vi "sub_log_fine-name.vi"() -> (3 "log path":string)   [LabVIEW 2019]
uses:
  logfile-name.vi
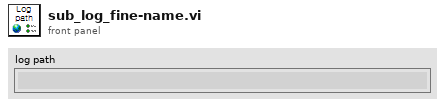
[diagram p1: front panel]
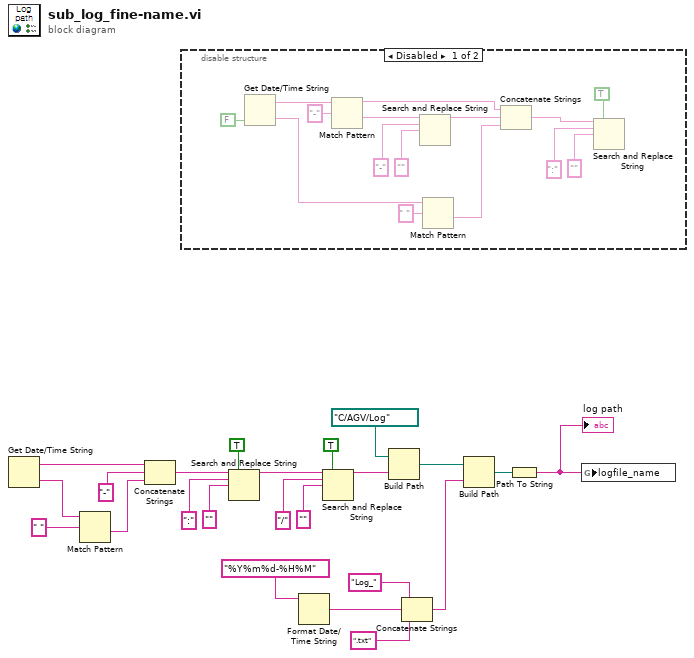
[diagram p0: block diagram]
diagram:
  n1 = Get Date/Time String() -> (date string=w11:string, time string=w17:string)  [unwired: 3 in]
  n2 = Match Pattern(string=w17, regular expression=" " ("정규식")) -> (after substring=w16:string)  [unwired: 1 in, 3 out]
  n3 = Concatenate Strings(w11, "-" ("정규식"), w16) -> (w12:string)
  n4 = disable-structure shown="Disabled" {
    frame Disabled {
      n5 = Get Date/Time String(want seconds? (F)=FALSE ("초 보이기? (거짓)")) -> (date string=w33:string, time string=w30:string)  [unwired: 2 in]
      n6 = Match Pattern(string=w33, regular expression="-" ("정규식")) -> (before substring=w24:string, after substring=w28:string)  [unwired: 1 in, 2 out]
      n7 = Search and Replace String(input string=w28, search string="-" ("검색 문자열"), replace string="" ("대체 문자열(\"\")")) -> (result string=w25:string)  [unwired: 5 in, 3 out]
      n8 = Match Pattern(string=w30, regular expression=" " ("정규식")) -> (after substring=w29:string)  [unwired: 1 in, 3 out]
      n9 = Concatenate Strings(w24, w25, w29) -> (w38:string)
      n10 = Search and Replace String(replace all?=TRUE ("모두 대체? (거짓)"), input string=w38, search string=":" ("검색 문자열"), replace string="" ("대체 문자열(\"\")")) -> ()  [unwired: 4 in, 4 out]
    }
    frame Enabled {
    }
  }
  n11 = Search and Replace String(replace all?=TRUE ("모두 대체? (거짓)"), input string=w12, search string=":" ("검색 문자열"), replace string="" ("대체 문자열(\"\")")) -> (result string=w2:string)  [unwired: 4 in, 3 out]
  n12 = Format Date/Time String(time format string (%c)="%Y%m%d-%H%M") -> (date/time string=w20:string)  [unwired: 2 in]
  n13 = Search and Replace String(replace all?=TRUE ("모두 대체? (거짓)"), input string=w2, search string="/" ("검색 문자열"), replace string="" ("대체 문자열(\"\")")) -> (result string=w1:string)  [unwired: 4 in, 3 out]
  n14 = Build Path(base path=path "C:/AGV/Log" ("베이스 경로"), name or relative path=w1) -> (appended path=w8:path)
  n15 = Concatenate Strings("Log_", w20, ".txt" ("문자열")) -> (w9:string)
  n16 = Build Path(base path=w8, name or relative path=w9) -> (appended path=w7:path)
  n17 = Path To String(path=w7) -> (string=w6:string)
  "log path" <- w6
  n18 = global write "logfile-name.vi" "logfile_name"(w6) -> ()
